vi "TL28 Reles Main.vi"() -> ()   [LabVIEW 2023]
uses:
  Controles/Boton_Gas.ctl
  Controles/Relevador.ctl
  Controles/Casos.ctl
  Controles/States_Read_Erds_Current.ctl
  Common/LabVIEW GEA2 Toolkit/GEA3/type defs/Source_Destination.ctl
  Common/LabVIEW GEA2 Toolkit/GEA3/type defs/ERD Read Data In.ctl
  Common/LabVIEW GEA2 Toolkit/GEA3/type defs/ERD Write Data In.ctl
  Common/LabVIEW GEA2 Toolkit/GEA3/type defs/Data Type.ctl
  Common/LabVIEW GEA2 Toolkit/GEA3/library/GEA2_Toolkit.lvlib
panel:
  out "CSV File Log Path":path
  in  "Start Graf":bool
  in  "Gas":T1
  in  "Eléctrica":T1
  in  "Stop Button":bool
  in  "Play Button":bool
  out "RL2":bool
  out "RL1":bool
  out "ELECTRICA":bool
  out "GAS":bool
  out "Pausa":bool
  out "Start":bool
  out "Dialogo":string
  out "Seconds":i16
  in  "Tab Control 2":enum32{"Configuracion", "Gráficas"}(tab)
  in  "Tab_Control":enum32{"ELÉCTRICA", "GAS"}(tab)
  in  "Tiempo RL1&RL2":i16=1 min=0 step=1
  in  "Tiempo RL2":i16=1 min=0 step=1
  in  "Tiempo apagado":i16=1 min=0 step=1
  in  "Tiempo RL1 ON":i16=1 min=0 step=1
  in  "Tiempo RL1 OFF":i16=1
  out "Graph":cluster{u32, u32, u32, u32, u32, u32}(graph)
  in  "Time adquisition (ms)":u32=100
  out "N.O":bool
  out "N.C":bool
  out "Tipo_Rele":i32
  in  "Rele N.C":T2
  in  "Rele N.O":T2
  out "Error Out":errorcluster
  in  "Index":u8=1 max=4 step=1
  in  "Exit":bool
  # "Relevadores"
  # "Definición de tiempos"
  # "Defina los tiempos"
  # "Defina los tiempos"
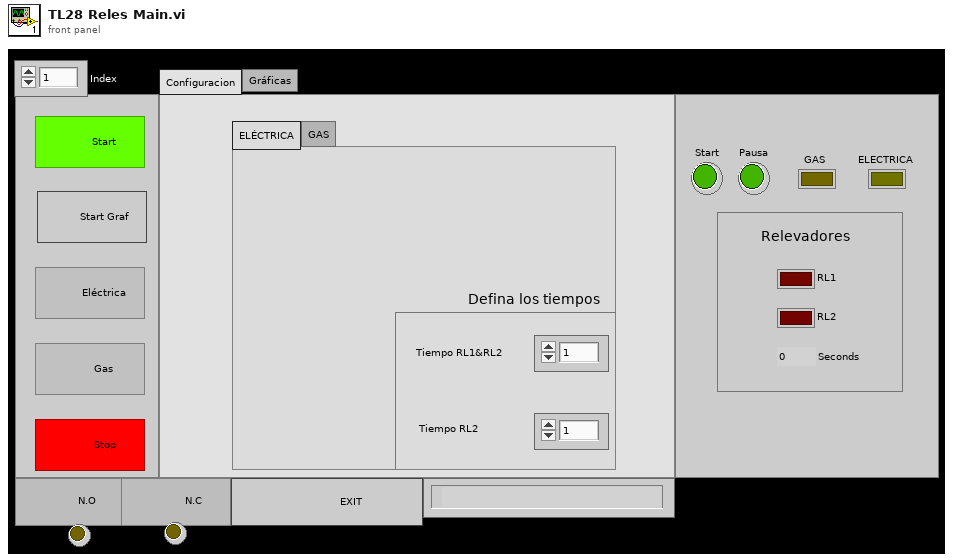
[diagram p1: front panel]
types:
  T1 = typedef "Boton_Gas.ctl" = bool
  T2 = typedef "Relevador.ctl" = bool
  T3 = typedef "States_Read_Erds_Current.ctl" = enum16{"Standby", "Read Erds", "Graph", "Save csv", "Pause"}
  T4 = typedef "Casos.ctl" = enum16{"Standby", "Seleccion", "Pausa", "RL1&RL2_Elect", "RL2_Elect", "OFF_Elect", "RL1_Gas", "OFF_Gas", "Seleccion NC", "Exit"}
  T5 = enum8{"Enabled", "Disabled", "Disabled and Grayed Out"}
  T6 = typedef "ERD Write Data In.ctl" = cluster{"ERD Number":u16, "Data Type":T7, "Data":string}
  T7 = typedef "Data Type.ctl" = enum16{"string", "boolean", "uint8_t", "uint16_t", "uint32_t", "uint64_t", "int8_t", "int16_t", "int32_t", "int64_t"}
  T8 = typedef "ERD Read Data In.ctl" = cluster{"ERD Number":u16, "Data Type":enum16{"string", "boolean", "uint8_t", "uint16_t", "uint32_t", "uint64_t", "int8_t", "int16_t", "int32_t", "int64_t"}}
  T9 = typedef "Source_Destination.ctl" = cluster{"Source":u8, "Destination":u8}
  T10 = typedef "ERD Read Data Out.ctl" = cluster{"ERD Number":u16, "Data":string}
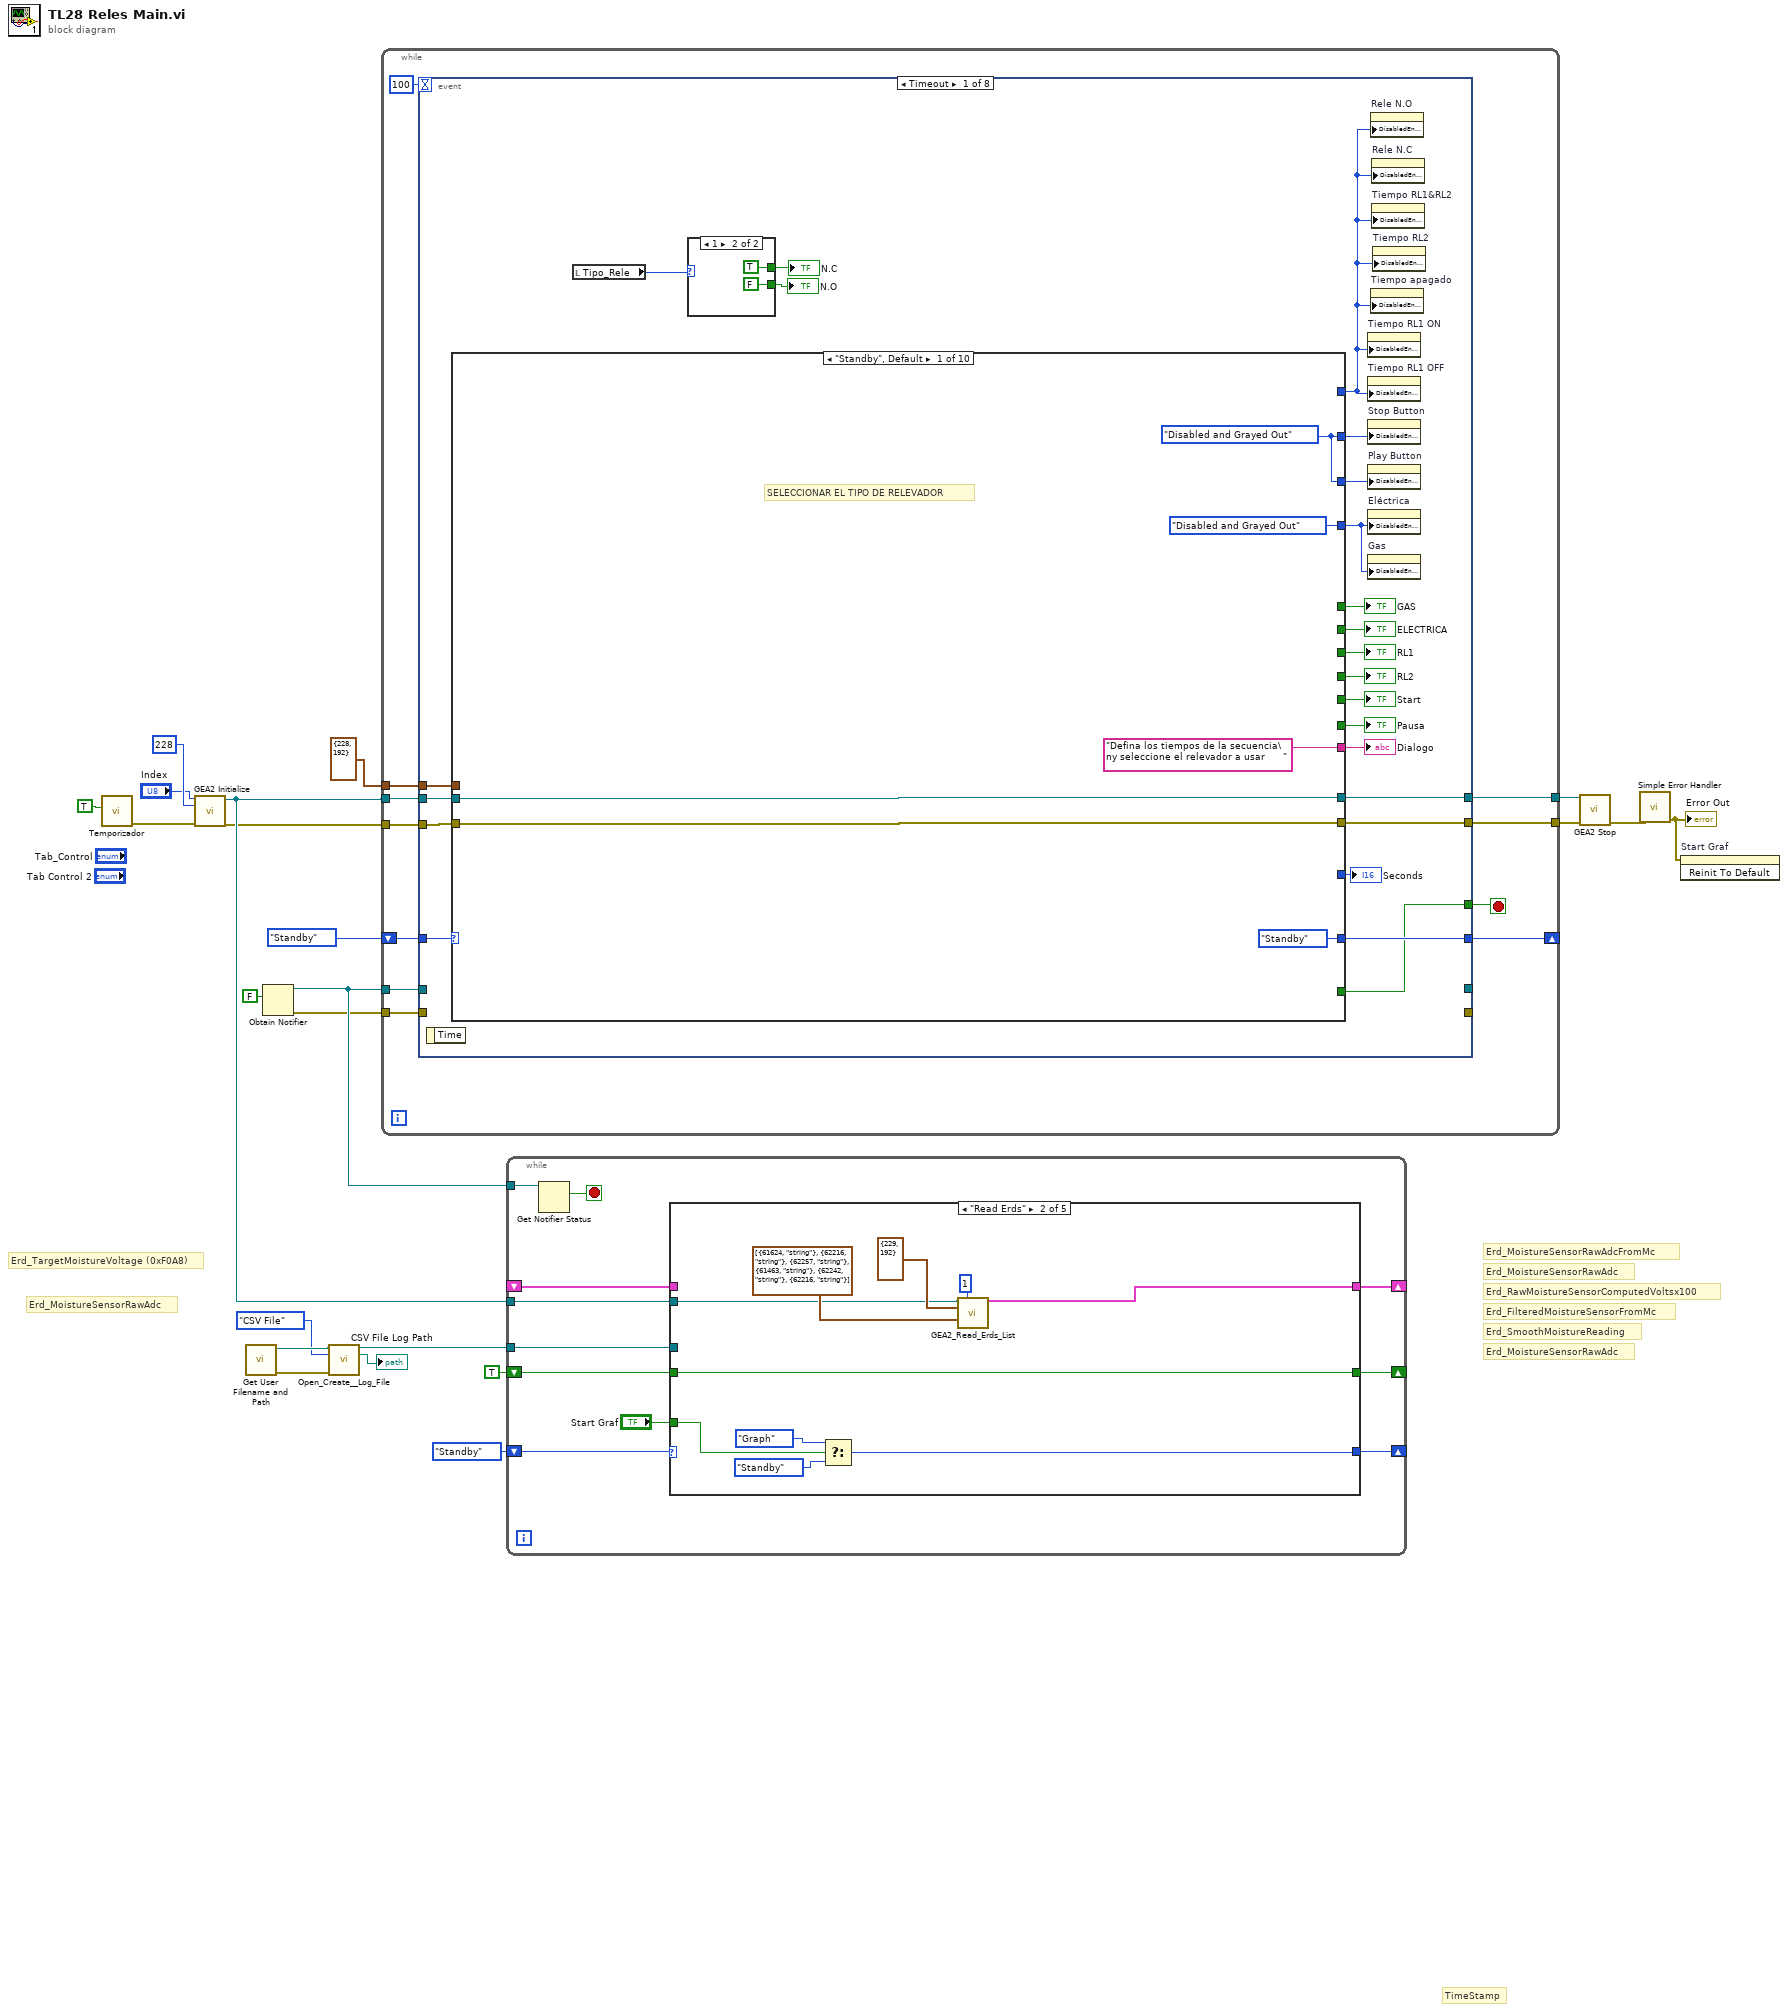
[diagram p0: block diagram]
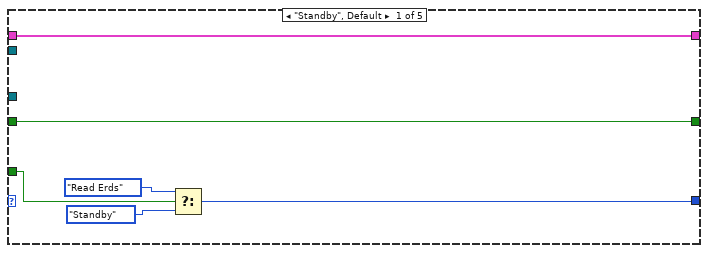
[diagram p2: hidden frame]
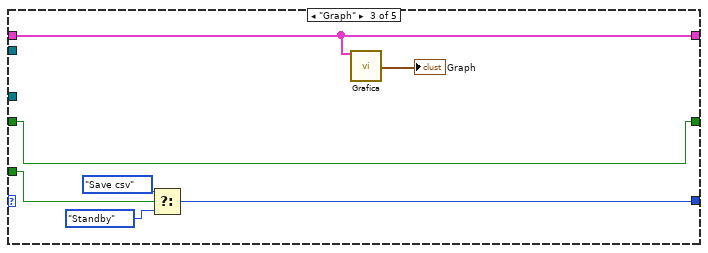
[diagram p3: hidden frame]
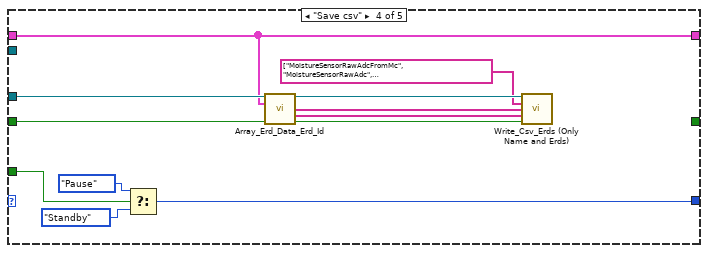
[diagram p4: hidden frame]
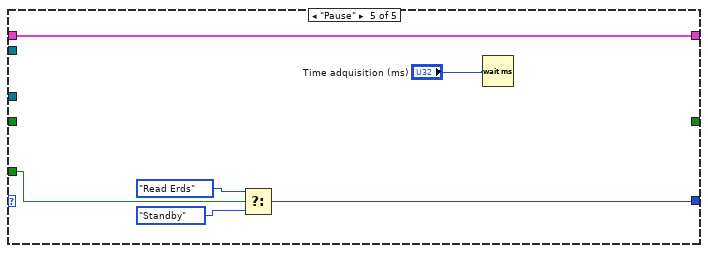
[diagram p5: hidden frame]
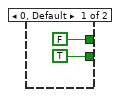
[diagram p6: hidden frame]
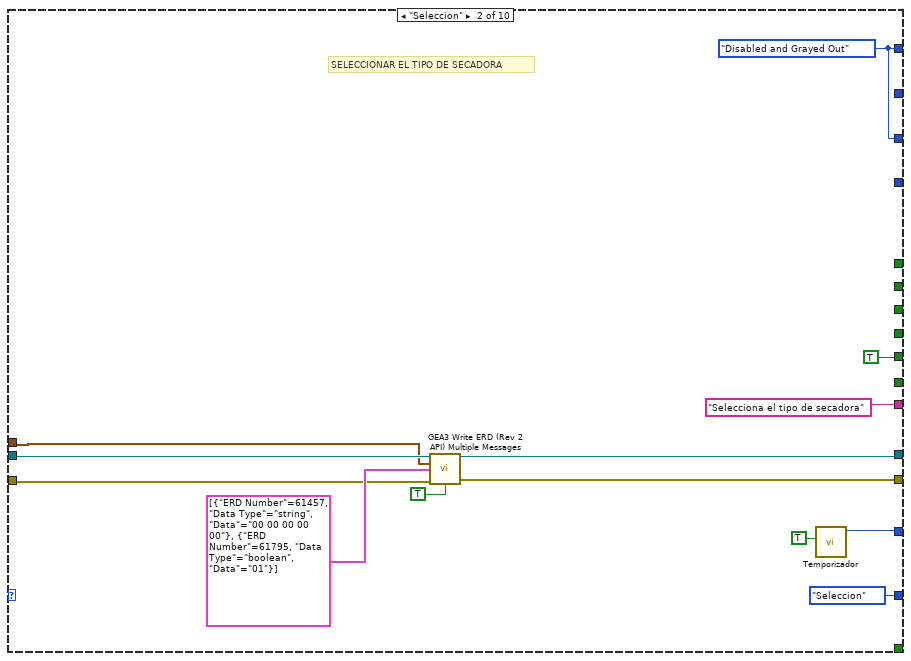
[diagram p7: hidden frame]
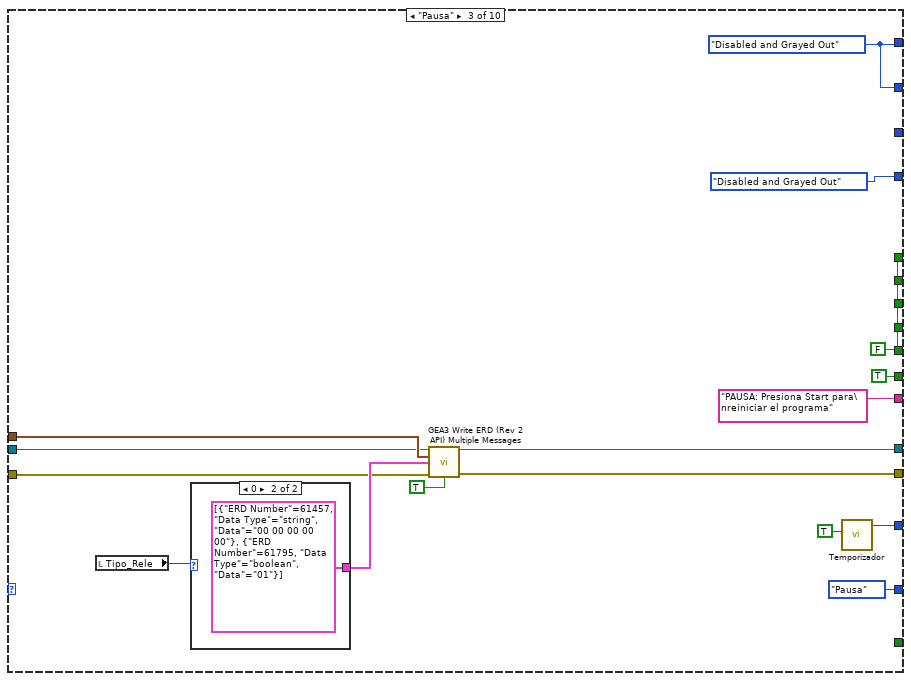
[diagram p8: hidden frame]
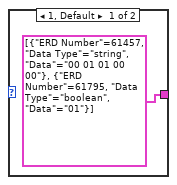
[diagram p9: hidden frame]
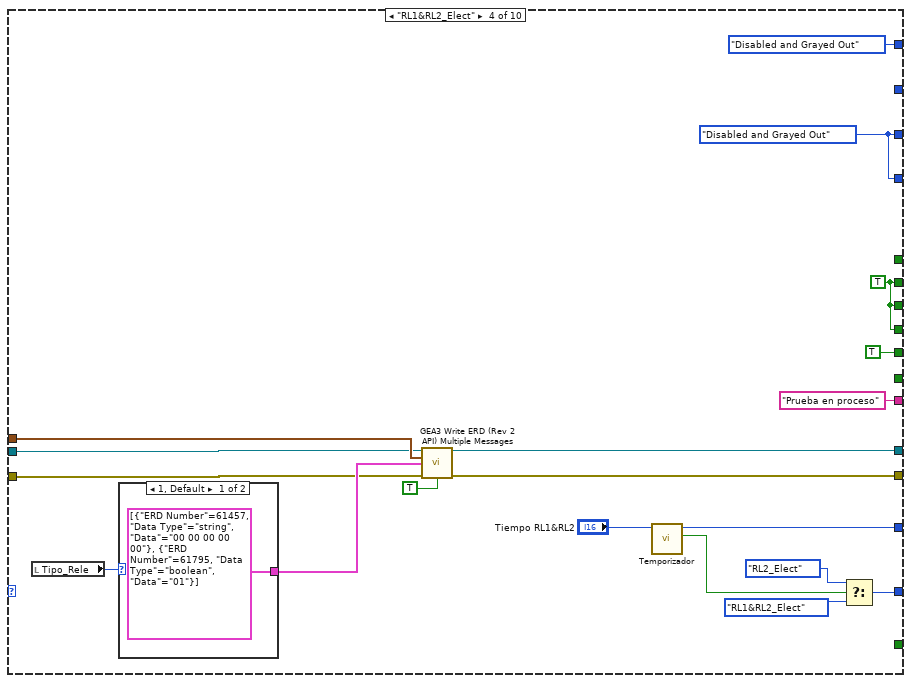
[diagram p10: hidden frame]
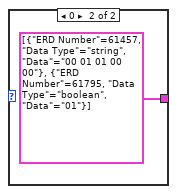
[diagram p11: hidden frame]
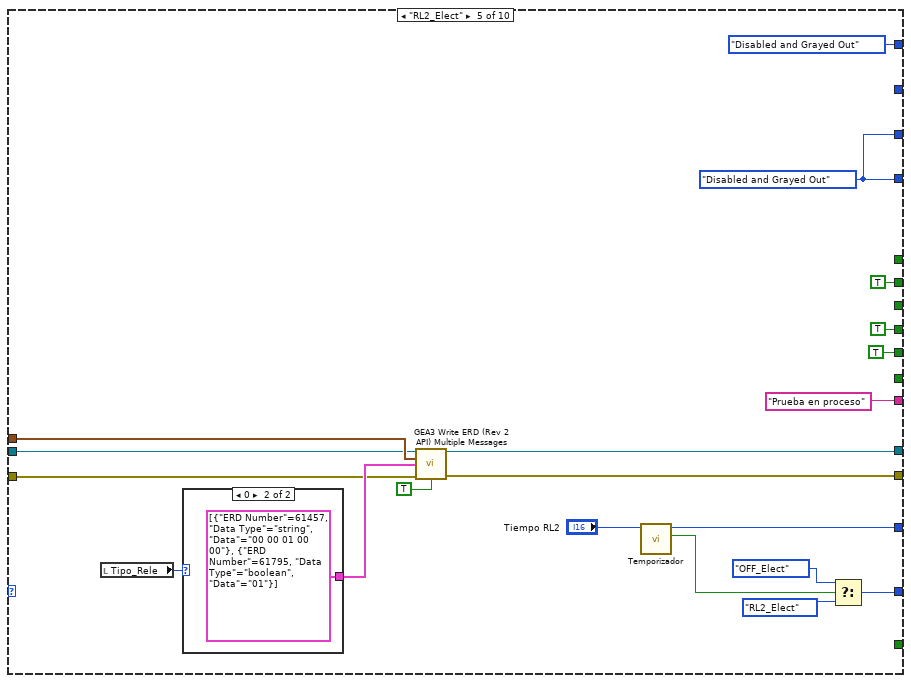
[diagram p12: hidden frame]
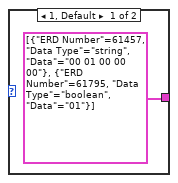
[diagram p13: hidden frame]
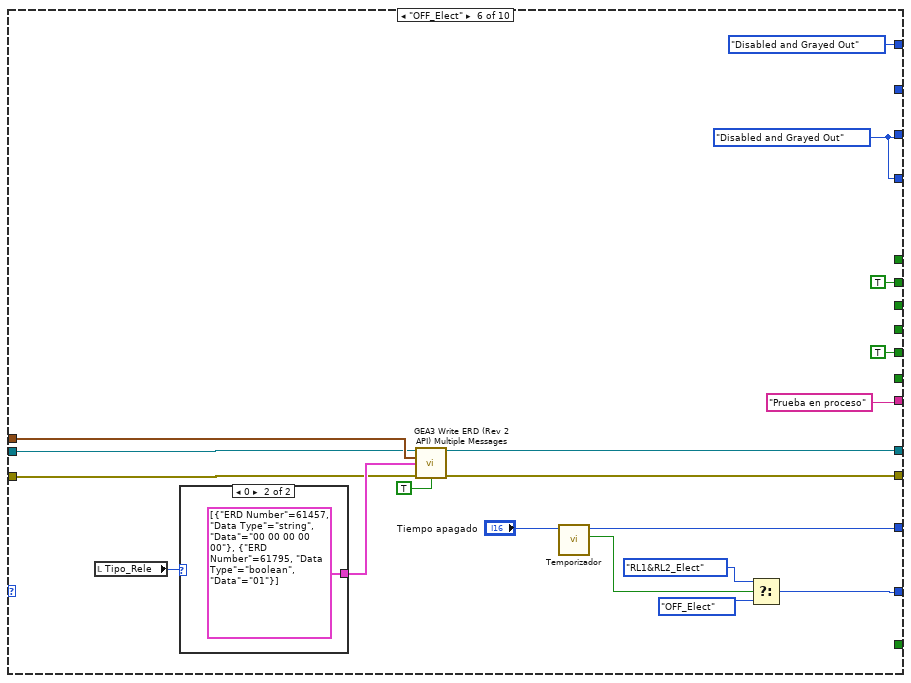
[diagram p14: hidden frame]
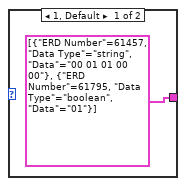
[diagram p15: hidden frame]
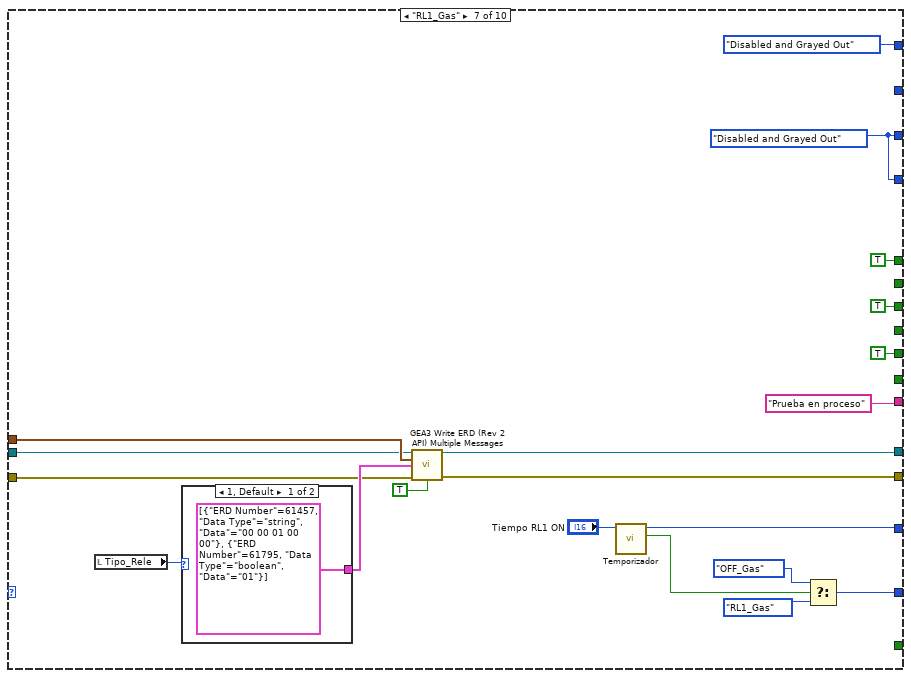
[diagram p16: hidden frame]
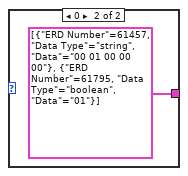
[diagram p17: hidden frame]
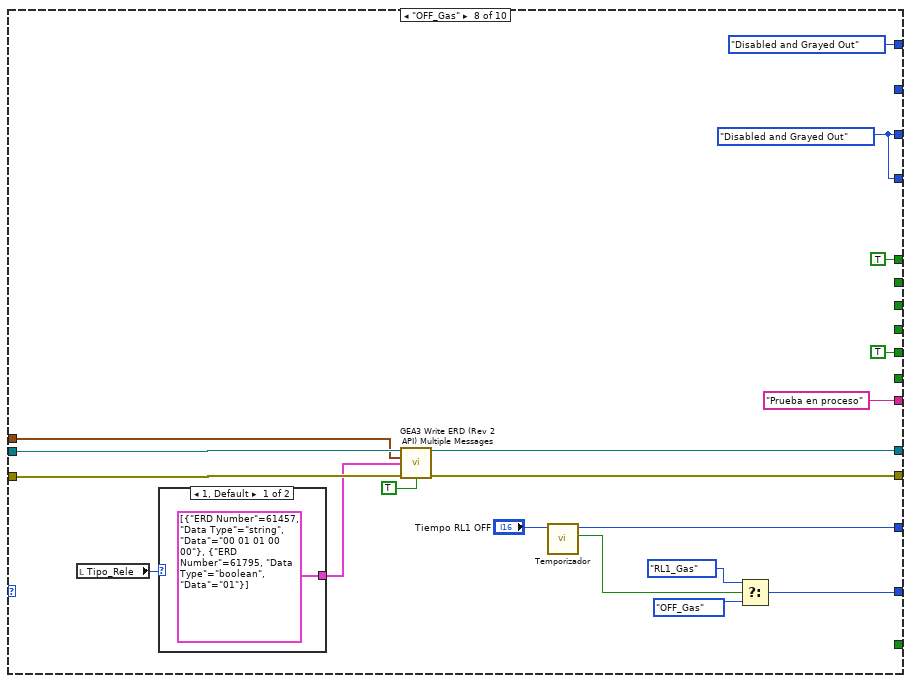
[diagram p18: hidden frame]
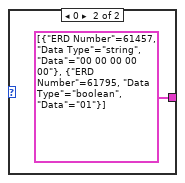
[diagram p19: hidden frame]
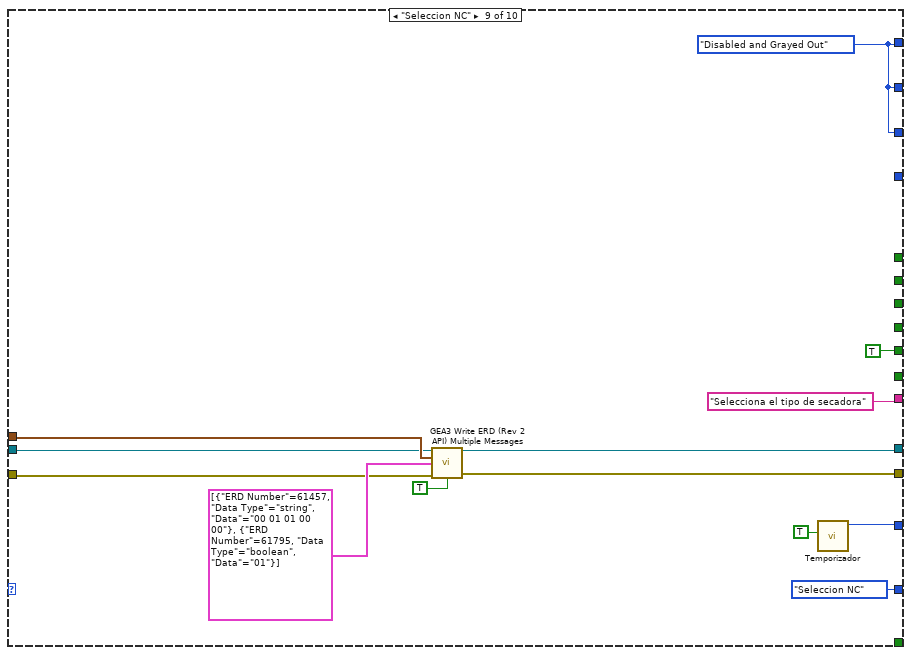
[diagram p20: hidden frame]
diagram:
  # "TimeStamp"
  # "Erd_MoistureSensorRawAdc"
  # "Erd_SmoothMoistureReading"
  # "Erd_FilteredMoistureSensorFromMc"
  # "Erd_RawMoistureSensorComputedVoltsx100"
  # "Erd_MoistureSensorRawAdc"
  # "Erd_MoistureSensorRawAdcFromMc"
  # "Erd_MoistureSensorRawAdc"
  # "Erd_TargetMoistureVoltage (0xF0A8)"
  n1 = call "Temporizador.vi"("Reset buton"=TRUE ("Reset")) -> ("error out"=w14:errorcluster)  [unwired: 8 in, 2 out]
  n2 = call "GEA2 Initialize.vi"("Board Index"="Index", "Source Address"=u8 228, "error in"=w14) -> ("GEA2 Reference Out"=w9:refnum<k24>, "error out"=w8:errorcluster)  [unwired: 10 in, 1 out]
  n3 = call "Get User Filename and Path.vi"() -> ("error out"=w7:errorcluster, "CSV File Path"=w6:path)  [unwired: 9 in, 1 out]
  n4 = Obtain Notifier(notification data type=FALSE) -> (notifier out=w11:refnum<notifier>, error out=w10:errorcluster)  [unwired: 3 in, 1 out]
  n5 = call "Open_Create__Log_File.vi"("File Path Control"=w6, "Enum"=enum16{"CSV File", "Text File"}."CSV File", "Error In"=w7) -> ("refnum out"=w3:refnum<file>, "File Path"=→"CSV File Log Path":path)  [unwired: 10 in, 1 out]
  n6 = while {
    shift-right: [w32] -> _
    shift-left: Casos."Standby" -> [w33]
    tunnel: w9 -> [w30]
    tunnel: w8 -> [w29]
    tunnel: cluster{"Source":u8, "Destination":u8} {"Source"=228, "Destination"=192} ("GEA Inputs") -> [w28]
    tunnel: [w27] -> w17
    tunnel: [w26] -> w16
    tunnel: w11 -> [w24]
    tunnel: w10 -> [w23]
    stop <- w25 stop-if-true
    n7 = event shown="[0] Timeout" {
      selector: _ -> [_ _ _ _ _ _ _ _]
      dyn-events: _ -> [_ _ _ _ _ _ _ _]
      timeout: 100 -> [_ _ _ _ _ _ _ _]
      tunnel: w33 -> [w56 _ _ _ _ _ _ _]
      tunnel: [w55 Casos."Standby" Casos."Pausa" Casos."RL1_Gas" Casos."RL1&RL2_Elect" Casos."Seleccion" Casos."Seleccion" Casos."Exit"] -> w32
      tunnel: [w54 _ _ _ _ _ _ _] -> w25
      tunnel: w30 -> [w45 w231 w234 w240 w248 w253 w257 w266]
      tunnel: w29 -> [w44 w230 w233 w239 w247 w252 w256 w265]
      tunnel: w28 -> [w43 _ _ w241 w249 _ _ _]
      tunnel: [w42 w231 w234 w238 w246 w253 w257 w266] -> w27
      tunnel: [w41 w230 w233 w237 w245 w252 w256 w265] -> w26
      tunnel: w24 -> [_ _ _ _ _ _ _ w263]
      tunnel: w23 -> [_ _ _ _ _ _ _ w262]
      tunnel: [_ _ _ _ _ _ _ w261] -> _
      tunnel: [_ _ _ _ _ _ _ w260] -> _
      event Timeout {
        n8 = event-data() -> ()  [unwired: 1 in, 1 out]
        n9 = case shown="\"Standby\", Default" w56 {
          tunnel: [Casos."Standby" Casos."Seleccion" Casos."Pausa" w111 w131 w154 w177 w198 Casos."Seleccion NC" _] -> w55
          tunnel: [_ _ _ _ _ _ _ _ _ TRUE] -> w54
          tunnel: [_ TRUE _ TRUE TRUE TRUE TRUE TRUE TRUE _] -> w53
          tunnel: ["Defina los tiempos de la secuencia\ny seleccione el relevador a usar      " "Selecciona el tipo de secadora" "PAUSA: Presiona Start para\nreiniciar el programa" "Prueba en proceso" "Prueba en proceso" "Prueba en proceso" "Prueba en proceso" "Prueba en proceso" "Selecciona el tipo de secadora" "Exit"] -> w52
          tunnel: [_ _ w93 w110 TRUE TRUE _ _ _ _] -> w51
          tunnel: [_ _ w93 _ _ _ TRUE TRUE _ _] -> w50
          tunnel: [_ _ TRUE _ _ _ _ _ _ _] -> w49
          tunnel: [_ _ _ w110 _ _ TRUE _ _ _] -> w48
          tunnel: [_ _ _ w110 TRUE _ _ _ _ _] -> w47
          tunnel: [_ w76 w83 w109 w130 w153 w176 w197 w206 _] -> w46
          tunnel: [_ w67 w81 T5."Disabled and Grayed Out" ("Disabled") T5."Disabled and Grayed Out" ("Disabled") T5."Disabled and Grayed Out" ("Disabled") T5."Disabled and Grayed Out" ("Disabled") T5."Disabled and Grayed Out" ("Disabled") w217 _] -> w37
          tunnel: w45 -> [w64 w71 w88 w103 w124 w147 w167 w192 w212 w222]
          tunnel: w44 -> [w63 w72 w87 w102 w123 w146 w166 w191 w211 w221]
          tunnel: w43 -> [_ w70 w89 w104 w125 w148 w168 w188 w213 w223]
          tunnel: [w64 w69 w86 w101 w122 w145 w165 w187 w210 w220] -> w42
          tunnel: [w63 w68 w85 w100 w121 w144 w164 w186 w209 w219] -> w41
          tunnel: [w61 _ w81 _ _ _ _ _ w217 _] -> w40
          tunnel: [w61 w67 _ w99 w120 w142 w163 w185 w217 _] -> w39
          tunnel: [T5."Disabled and Grayed Out" ("Disabled") _ T5."Disabled and Grayed Out" ("Disabled") w99 w120 w142 w163 w185 _ _] -> w38
          frame "Standby", Default {
            w61 = T5."Disabled and Grayed Out" ("Disabled")
            # "SELECCIONAR EL TIPO DE RELEVADOR"
          }
          frame "Seleccion" {
            w67 = T5."Disabled and Grayed Out" ("Disabled")
            # "SELECCIONAR EL TIPO DE SECADORA"
            n10 = call "GEA3 Write ERD (Rev 2 API) Multiple Messages.vi"("GEA2 Reference In"=w71, "GEA Inputs"=w70, "Write ERD List"=T6[] [{"ERD Number"=61457, "Data Type"=enum."string", "Data"="00 00 00 00 00"}, {"ERD Number"=61795, "Data Type"=enum."boolean", "Data"="01"}], "Error In"=w72, "Verify ERD Response?"=TRUE) -> ("GEA2 Reference Out"=w69:refnum<k24>, "Error Out"=w68:errorcluster)  [unwired: 8 in, 1 out]
            n11 = call "Temporizador.vi"("Reset buton"=TRUE ("Reset")) -> ("Sec"=w76:i16)  [unwired: 8 in, 2 out]
          }
          frame "Pausa" {
            w81 = T5."Disabled and Grayed Out" ("Disabled")
            w93 = FALSE
            n12 = local read "Tipo_Rele"() -> (w80:i32)
            n13 = case shown="0" w80 {
              tunnel: [T6[] [{"ERD Number"=61457, "Data Type"=enum."string", "Data"="00 01 01 00 00"}, {"ERD Number"=61795, "Data Type"=enum."boolean", "Data"="01"}] T6[] [{"ERD Number"=61457, "Data Type"=enum."string", "Data"="00 00 00 00 00"}, {"ERD Number"=61795, "Data Type"=enum."boolean", "Data"="01"}]] -> w91
              frame 1, Default {
              }
              frame 0 {
              }
            }
            n14 = call "GEA3 Write ERD (Rev 2 API) Multiple Messages.vi"("GEA2 Reference In"=w88, "GEA Inputs"=w89, "Write ERD List"=w91, "Error In"=w87, "Verify ERD Response?"=TRUE) -> ("GEA2 Reference Out"=w86:refnum<k24>, "Error Out"=w85:errorcluster)  [unwired: 8 in, 1 out]
            n15 = call "Temporizador.vi"("Reset buton"=TRUE) -> ("Sec"=w83:i16)  [unwired: 8 in, 2 out]
          }
          frame "RL1&RL2_Elect" {
            w110 = TRUE
            w99 = T5."Disabled and Grayed Out" ("Disabled")
            n16 = local read "Tipo_Rele"() -> (w98:i32)
            n17 = case shown="1, Default" w98 {
              tunnel: [T6[] [{"ERD Number"=61457, "Data Type"=enum."string", "Data"="00 00 00 00 00"}, {"ERD Number"=61795, "Data Type"=enum."boolean", "Data"="01"}] T6[] [{"ERD Number"=61457, "Data Type"=enum."string", "Data"="00 01 01 00 00"}, {"ERD Number"=61795, "Data Type"=enum."boolean", "Data"="01"}]] -> w106
              frame 1, Default {
              }
              frame 0 {
              }
            }
            n18 = call "GEA3 Write ERD (Rev 2 API) Multiple Messages.vi"("GEA2 Reference In"=w103, "GEA Inputs"=w104, "Write ERD List"=w106, "Error In"=w102, "Verify ERD Response?"=TRUE) -> ("GEA2 Reference Out"=w101:refnum<k24>, "Error Out"=w100:errorcluster)  [unwired: 8 in, 1 out]
            n19 = call "Temporizador.vi"("Set Time"="Tiempo RL1&RL2") -> ("Next"=w114:bool, "Sec"=w109:i16)  [unwired: 8 in, 1 out]
            n20 = Select(t=Casos."RL2_Elect", s=w114, f=Casos."RL1&RL2_Elect") -> (s? t:f=w111:T4)
          }
          frame "RL2_Elect" {
            w120 = T5."Disabled and Grayed Out" ("Disabled")
            n21 = local read "Tipo_Rele"() -> (w119:i32)
            n22 = case shown="0" w119 {
              tunnel: [T6[] [{"ERD Number"=61457, "Data Type"=enum."string", "Data"="00 01 00 00 00"}, {"ERD Number"=61795, "Data Type"=enum."boolean", "Data"="01"}] T6[] [{"ERD Number"=61457, "Data Type"=enum."string", "Data"="00 00 01 00 00"}, {"ERD Number"=61795, "Data Type"=enum."boolean", "Data"="01"}]] -> w127
              frame 1, Default {
              }
              frame 0 {
              }
            }
            n23 = call "GEA3 Write ERD (Rev 2 API) Multiple Messages.vi"("GEA2 Reference In"=w124, "GEA Inputs"=w125, "Write ERD List"=w127, "Error In"=w123, "Verify ERD Response?"=TRUE) -> ("GEA2 Reference Out"=w122:refnum<k24>, "Error Out"=w121:errorcluster)  [unwired: 8 in, 1 out]
            n24 = call "Temporizador.vi"("Set Time"="Tiempo RL2") -> ("Next"=w136:bool, "Sec"=w130:i16)  [unwired: 8 in, 1 out]
            n25 = Select(t=Casos."OFF_Elect", s=w136, f=Casos."RL2_Elect") -> (s? t:f=w131:T4)
          }
          frame "OFF_Elect" {
            w142 = T5."Disabled and Grayed Out" ("Disabled")
            n26 = local read "Tipo_Rele"() -> (w141:i32)
            n27 = case shown="0" w141 {
              tunnel: [T6[] [{"ERD Number"=61457, "Data Type"=enum."string", "Data"="00 01 01 00 00"}, {"ERD Number"=61795, "Data Type"=enum."boolean", "Data"="01"}] T6[] [{"ERD Number"=61457, "Data Type"=enum."string", "Data"="00 00 00 00 00"}, {"ERD Number"=61795, "Data Type"=enum."boolean", "Data"="01"}]] -> w150
              frame 1, Default {
              }
              frame 0 {
              }
            }
            n28 = call "GEA3 Write ERD (Rev 2 API) Multiple Messages.vi"("GEA2 Reference In"=w147, "GEA Inputs"=w148, "Write ERD List"=w150, "Error In"=w146, "Verify ERD Response?"=TRUE) -> ("GEA2 Reference Out"=w145:refnum<k24>, "Error Out"=w144:errorcluster)  [unwired: 8 in, 1 out]
            n29 = call "Temporizador.vi"("Set Time"="Tiempo apagado") -> ("Next"=w158:bool, "Sec"=w153:i16)  [unwired: 8 in, 1 out]
            n30 = Select(t=Casos."RL1&RL2_Elect", s=w158, f=Casos."OFF_Elect") -> (s? t:f=w154:T4)
          }
          frame "RL1_Gas" {
            w163 = T5."Disabled and Grayed Out" ("Disabled")
            n31 = local read "Tipo_Rele"() -> (w162:i32)
            n32 = case shown="1, Default" w162 {
              tunnel: [T6[] [{"ERD Number"=61457, "Data Type"=enum."string", "Data"="00 00 01 00 00"}, {"ERD Number"=61795, "Data Type"=enum."boolean", "Data"="01"}] T6[] [{"ERD Number"=61457, "Data Type"=enum."string", "Data"="00 01 00 00 00"}, {"ERD Number"=61795, "Data Type"=enum."boolean", "Data"="01"}]] -> w170
              frame 1, Default {
              }
              frame 0 {
              }
            }
            n33 = call "GEA3 Write ERD (Rev 2 API) Multiple Messages.vi"("GEA2 Reference In"=w167, "GEA Inputs"=w168, "Write ERD List"=w170, "Error In"=w166, "Verify ERD Response?"=TRUE) -> ("GEA2 Reference Out"=w165:refnum<k24>, "Error Out"=w164:errorcluster)  [unwired: 8 in, 1 out]
            n34 = call "Temporizador.vi"("Set Time"="Tiempo RL1 ON") -> ("Next"=w180:bool, "Sec"=w176:i16)  [unwired: 8 in, 1 out]
            n35 = Select(t=Casos."OFF_Gas", s=w180, f=Casos."RL1_Gas") -> (s? t:f=w177:T4)
          }
          frame "OFF_Gas" {
            w185 = T5."Disabled and Grayed Out" ("Disabled")
            n36 = local read "Tipo_Rele"() -> (w184:i32)
            n37 = case shown="1, Default" w184 {
              tunnel: [T6[] [{"ERD Number"=61457, "Data Type"=enum."string", "Data"="00 01 01 00 00"}, {"ERD Number"=61795, "Data Type"=enum."boolean", "Data"="01"}] T6[] [{"ERD Number"=61457, "Data Type"=enum."string", "Data"="00 00 00 00 00"}, {"ERD Number"=61795, "Data Type"=enum."boolean", "Data"="01"}]] -> w190
              frame 1, Default {
              }
              frame 0 {
              }
            }
            n38 = call "GEA3 Write ERD (Rev 2 API) Multiple Messages.vi"("GEA2 Reference In"=w192, "GEA Inputs"=w188, "Write ERD List"=w190, "Error In"=w191, "Verify ERD Response?"=TRUE) -> ("GEA2 Reference Out"=w187:refnum<k24>, "Error Out"=w186:errorcluster)  [unwired: 8 in, 1 out]
            n39 = call "Temporizador.vi"("Set Time"="Tiempo RL1 OFF") -> ("Next"=w201:bool, "Sec"=w197:i16)  [unwired: 8 in, 1 out]
            n40 = Select(t=Casos."RL1_Gas", s=w201, f=Casos."OFF_Gas") -> (s? t:f=w198:T4)
          }
          frame "Seleccion NC" {
            w217 = T5."Disabled and Grayed Out" ("Disabled")
            n41 = call "GEA3 Write ERD (Rev 2 API) Multiple Messages.vi"("GEA2 Reference In"=w212, "GEA Inputs"=w213, "Write ERD List"=T6[] [{"ERD Number"=61457, "Data Type"=enum."string", "Data"="00 01 01 00 00"}, {"ERD Number"=61795, "Data Type"=enum."boolean", "Data"="01"}], "Error In"=w211, "Verify ERD Response?"=TRUE) -> ("GEA2 Reference Out"=w210:refnum<k24>, "Error Out"=w209:errorcluster)  [unwired: 8 in, 1 out]
            n42 = call "Temporizador.vi"("Reset buton"=TRUE ("Reset")) -> ("Sec"=w206:i16)  [unwired: 8 in, 2 out]
          }
          frame "Exit" {
            n43 = local read "Tipo_Rele"() -> (w218:i32)
            n44 = case shown="1, Default" w218 {
              tunnel: [T6[] [{"ERD Number"=61457, "Data Type"=enum."string", "Data"="00 01 01 00 00"}, {"ERD Number"=61795, "Data Type"=enum."boolean", "Data"="00"}] T6[] [{"ERD Number"=61457, "Data Type"=enum."string", "Data"="00 00 00 00 00"}, {"ERD Number"=61795, "Data Type"=enum."boolean", "Data"="00"}]] -> w225
              frame 1, Default {
              }
              frame 0 {
              }
            }
            n45 = call "GEA3 Write ERD (Rev 2 API) Multiple Messages.vi"("GEA2 Reference In"=w222, "GEA Inputs"=w223, "Write ERD List"=w225, "Error In"=w221, "Verify ERD Response?"=FALSE) -> ("GEA2 Reference Out"=w220:refnum<k24>, "Error Out"=w219:errorcluster)  [unwired: 8 in, 1 out]
          }
        }
        "Start" <- w53
        "Dialogo" <- w52
        "ELECTRICA" <- w51
        "GAS" <- w50
        "Pausa" <- w49
        "RL1" <- w48
        "RL2" <- w47
        "Seconds" <- w46
        n46 = local read "Tipo_Rele"() -> (w36:i32)
        n47 = case shown="1" w36 {
          tunnel: [FALSE TRUE] -> w35
          tunnel: [TRUE FALSE] -> w34
          frame 0, Default {
          }
          frame 1 {
          }
        }
        "N.C" <- w35
        "N.O" <- w34
        n48 = property on="Tiempo RL1 ON" class="DigNum (strict)"("DisabledEnum"=w37) -> ()  [unwired: 2 in, 2 out]
        n49 = property on="Tiempo RL1 OFF" class="DigNum (strict)"("DisabledEnum"=w37) -> ()  [unwired: 2 in, 2 out]
        n50 = property on="Stop Button" class="Bool"("DisabledEnum"=w40) -> ()  [unwired: 2 in, 2 out]
        n51 = property on="Play Button" class="Bool"("DisabledEnum"=w39) -> ()  [unwired: 2 in, 2 out]
        n52 = property on="Eléctrica" class="Bool"("DisabledEnum"=w38) -> ()  [unwired: 2 in, 2 out]
        n53 = property on="Gas" class="Bool"("DisabledEnum"=w38) -> ()  [unwired: 2 in, 2 out]
        n54 = property on="Rele N.O" class="Bool"("DisabledEnum"=w37) -> ()  [unwired: 2 in, 2 out]
        n55 = property on="Tiempo apagado" class="DigNum (strict)"("DisabledEnum"=w37) -> ()  [unwired: 2 in, 2 out]
        n56 = property on="Rele N.C" class="Bool"("DisabledEnum"=w37) -> ()  [unwired: 2 in, 2 out]
        n57 = property on="Tiempo RL1&RL2" class="DigNum (strict)"("DisabledEnum"=w37) -> ()  [unwired: 2 in, 2 out]
        n58 = property on="Tiempo RL2" class="DigNum (strict)"("DisabledEnum"=w37) -> ()  [unwired: 2 in, 2 out]
      }
      event "Play Button": Value Change {
        n59 = event-data() -> ()  [unwired: 1 in, 1 out]
      }
      event "Stop Button": Value Change {
        n60 = event-data() -> ()  [unwired: 1 in, 1 out]
      }
      event Value Change {
        n61 = event-data() -> ()  [unwired: 1 in, 1 out]
        n62 = call "GEA3 Write ERD (Rev 2 API) Multiple Messages.vi"("GEA2 Reference In"=w240, "GEA Inputs"=w241, "Write ERD List"=T6[] [{"ERD Number"=61795, "Data Type"=enum."boolean", "Data"="01"}], "Error In"=w239, "Verify ERD Response?"=FALSE) -> ("GEA2 Reference Out"=w238:refnum<k24>, "Error Out"=w237:errorcluster)  [unwired: 8 in, 1 out]
      }
      event Value Change {
        n63 = event-data() -> ()  [unwired: 1 in, 1 out]
        n64 = call "GEA3 Write ERD (Rev 2 API) Multiple Messages.vi"("GEA2 Reference In"=w248, "GEA Inputs"=w249, "Write ERD List"=T6[] [{"ERD Number"=61795, "Data Type"=enum."boolean", "Data"="01"}], "Error In"=w247, "Verify ERD Response?"=FALSE) -> ("GEA2 Reference Out"=w246:refnum<k24>, "Error Out"=w245:errorcluster)  [unwired: 8 in, 1 out]
      }
      event Value Change {
        n65 = event-data() -> ()  [unwired: 1 in, 1 out]
        "Tipo_Rele" <- 0 ("Tipo_Rele")
      }
      event Value Change {
        n66 = event-data() -> ()  [unwired: 1 in, 1 out]
        n67 = local write "Tipo_Rele"(1 ("Tipo_Rele")) -> ()
      }
      event "Exit": Value Change {
        n68 = event-data() -> ()  [unwired: 1 in, 1 out]
        n69 = Send Notification(notification=TRUE, notifier=w263, error in (no error)=w262) -> (notifier out=w261:refnum<notifier>, error out=w260:errorcluster)
      }
    }
  }
  n70 = while {
    shift-right: [w277] -> _
    shift-left: States_Read_Erds_Current."Standby" -> [w275]
    tunnel: w11 -> [w276]
    shift-right: [w273] -> _
    shift-left: _ -> [w272]
    tunnel: w9 -> [w271]
    tunnel: w3 -> [w270]
    shift-right: [w268] -> _
    shift-left: TRUE ("Write Header ? In") -> [w269]
    stop <- w274 stop-if-true
    n71 = Get Notifier Status(notifier=w276) -> (current notification=w274:bool)  [unwired: 1 in, 4 out]
    n72 = case shown="\"Read Erds\"" w275 {
      tunnel: "Start Graf" -> [w284 w292 w299 w309 w315]
      tunnel: [w282 w291 w298 w308 w314] -> w277
      tunnel: [w280 w286 w296 w305 w313] -> w273
      tunnel: w272 -> [w280 _ w296 w305 w313]
      tunnel: w271 -> [_ w288 _ _ _]
      tunnel: w270 -> [_ _ _ w307 _]
      tunnel: w269 -> [w279 w287 w297 w303 _]
      tunnel: [w279 w287 w297 _ _] -> w268
      frame "Standby", Default {
        n73 = Select(t=States_Read_Erds_Current."Read Erds", s=w284, f=States_Read_Erds_Current."Standby") -> (s? t:f=w282:T3)
      }
      frame "Read Erds" {
        n74 = Select(t=States_Read_Erds_Current."Graph", s=w292, f=States_Read_Erds_Current."Standby") -> (s? t:f=w291:T3)
        n75 = call "GEA2_Read_Erds_List.vi"(".NET Refnum in"=w288, "# of Iterations (Should be 2 except JL)"=1, "GEA Inputs"=T9 {"Source"=229, "Destination"=192}, "Read ERD List MC"=T8[] [{"ERD Number"=61624, "Data Type"=enum."string"}, {"ERD Number"=62216, "Data Type"=enum."string"}, {"ERD Number"=62257, "Data Type"=enum."string"}, {"ERD Number"=61463, "Data Type"=enum."string"}, {"ERD Number"=62242, "Data Type"=enum."string"}, {"ERD Number"=62216, "Data Type"=enum."string"}]) -> ("ERD Data Out out"=w286:T10[])  [unwired: 10 in, 1 out]
      }
      frame "Graph" {
        n76 = Select(t=States_Read_Erds_Current."Save csv", s=w299, f=States_Read_Erds_Current."Standby") -> (s? t:f=w298:T3)
        n77 = call "Grafica.vi"("ERD Data Out out"=w296) -> ("Graph"=→"Graph":cluster{u32, u32, u32, u32, u32, u32})  [unwired: 14 in]
      }
      frame "Save csv" {
        n78 = Select(t=States_Read_Erds_Current."Pause", s=w309, f=States_Read_Erds_Current."Standby") -> (s? t:f=w308:T3)
        n79 = call "Array_Erd_Data_Erd_Id.vi"("ERD Data Out out"=w305) -> ("Array_Erd_Number"=w302:string[], "Array_Erd_Data"=w304:string[])  [unwired: 13 in]
        n80 = call "Write_Csv_Erds (Only Name and Erds).vi"("Refnum_In_Csv"=w307, "ERD Name Array In"=string[] ["MoistureSensorRawAdcFromMc", "MoistureSensorRawAdc", "RawMoistureSensorComputedVoltsx100", "FilteredMoistureSensorFromMc", "SmoothMoistureReading", "MoistureSensorRawAdc"], "ERD Number Array In"=w302, "Data_Erd_Read"=w304, "Write Header ? In"=w303) -> ()  [unwired: 11 in]
      }
      frame "Pause" {
        n81 = Select(t=States_Read_Erds_Current."Read Erds", s=w315, f=States_Read_Erds_Current."Standby") -> (s? t:f=w314:T3)
        n82 = Wait (ms)(milliseconds to wait="Time adquisition (ms)") -> ()  [unwired: 1 out]
      }
    }
  }
  n83 = call "GEA2 Stop.vi"("GEA2 Reference In"=w17, "Error In"=w16) -> ("Error Out"=w18:errorcluster)  [unwired: 13 in]
  n84 = call <vilib>:"Simple Error Handler.vi"("error in (no error)"=w18) -> ("error out"=w1:errorcluster)  [unwired: 4 in, 4 out]
  "Error Out" <- w1
  n85 = invoke on="Start Graf" class="Bool (strict)" method="Reinit To Default"(error in=w1) -> ()  [unwired: 2 in, 3 out]
